vi "Bring Up.vi"(8 "error in (no error)":errorcluster, 11 "Assembler in":refnum<class "Assembler.lvclass">) -> (0 "error out":errorcluster, 3 "Assembler out":refnum<class "Assembler.lvclass">)   [LabVIEW 2016, in "CLD Exam - Car Wash.lvlib" / "Assembler.lvclass"]
uses:
  Assembler.lvclass
  D:/Repos/Stream/software/Actor/Actor Class/Ancestral Actor.lvclass
  Actor/Actor Class/Ancestral Actor.lvclass/Ancestral Actor.ctl
  Assembler.lvclass/Assembler.ctl
  Mediator/Classes/Message Broker Interface Ref/Message Broker Interface Ref.lvclass
  D:/Repos/Stream/software/Mediator/Classes/Message Broker Interface/Message Broker Interface.lvclass
  Car Position Simulator/Car Position Simulator.lvclass
  Car Wash Console/Car Wash Console.lvclass
  Car Wash Display/Car Wash Display.lvclass
  Car Wash Station Sequencer/Car Wash Station Sequencer.lvclass
  Actor/Actor Class/Ancestral Actor.lvclass
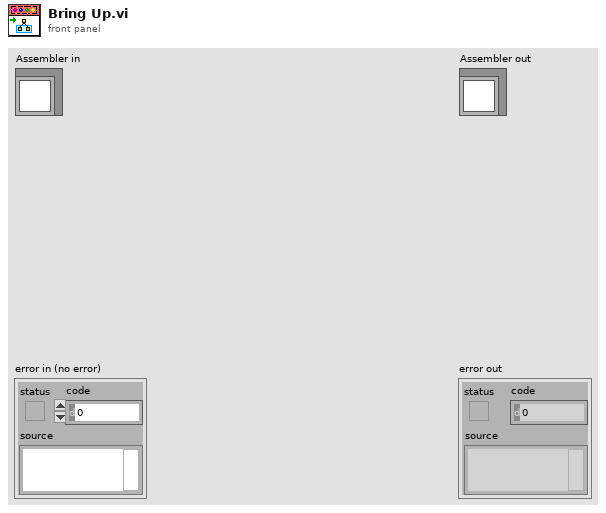
[diagram p1: front panel]
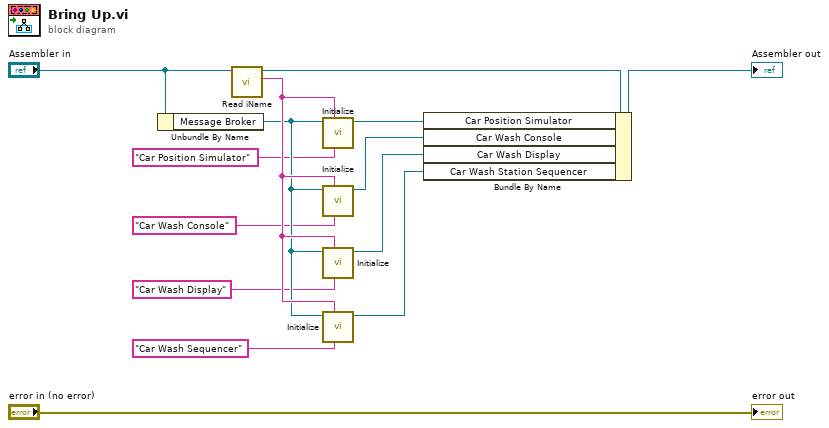
[diagram p0: block diagram]
diagram:
  n1 = Unbundle By Name("Assembler in") -> ("Message Broker"=w11:refnum<class "Message Broker Interface Ref.lvclass">)
  n2 = call "Read iName.vi"("Ancestral Actor in"="Assembler in") -> ("iName"=w12:string, "Ancestral Actor out"=w6:refnum<class "Assembler.lvclass">)  [unwired: 8 in, 1 out]
  n3 = call "Initialize.vi"("Actor Name"="Car Position Simulator", "Host Name"=w12, "Message Broker Interface"=w11) -> ("Car Position Simulator out"=w4:refnum<class "Car Position Simulator.lvclass">)  [unwired: 7 in, 1 out]
  n4 = call "Initialize.vi"("Actor Name"="Car Wash Console", "Host Name"=w12, "Message Broker Interface"=w11) -> ("Car Wash Console out"=w3:refnum<class "Car Wash Console.lvclass">)  [unwired: 7 in, 1 out]
  n5 = call "Initialize.vi"("Actor Name"="Car Wash Display", "Host Name"=w12, "Message Broker Interface"=w11) -> ("Car Wash Display out"=w2:refnum<class "Car Wash Display.lvclass">)  [unwired: 7 in, 1 out]
  n6 = call "Initialize.vi"("Actor Name"="Car Wash Sequencer", "Host Name"=w12, "Message Broker Interface"=w11) -> ("Car Wash Station Sequencer out"=w1:refnum<class "Car Wash Station Sequencer.lvclass">)  [unwired: 7 in, 1 out]
  n7 = Bundle By Name(cluster=w6, "Car Position Simulator"=w4, "Car Wash Console"=w3, "Car Wash Display"=w2, "Car Wash Station Sequencer"=w1) -> (→"Assembler out":refnum<class "Assembler.lvclass">)
  "error out" <- "error in (no error)"
